vi "Demo for Ba RT.vi"(4 "Source:Advanced:Source Delay":dbl=4e-05 format="%#_6p", 5 "Source:Transient Response":i32(ring)=1039 items=["Slow"=1041, "Normal"=1038, "Fast"=1039, "Custom"=1042], 7 "Measurement:Sense":i32(ring)=1009 items=["Local"=1008, "Remote"=1009], 8 "channels":string="0", 9 "Current":dbl=0.4 format="%#_6p", 10 "Voltage":dbl=0.6 format="%#_6p", 11 "resource name":refnum<k15>="SMU") -> (2 "R":dbl=1.3110205691793813e-05 format="%#_8p")   [LabVIEW 2019]
uses:
  <instrlib>/niDCPower/nidcpower.llb/niDCPower Wait For Event - Event.ctl
  <vilib>/ptbypt/NI_PtbyPt.lvlib
panel:
  in  "Measurement:Aperture":dbl=0.0833333333333333 format="%#_6p"
  out "error out":errorcluster
  out "current measurements":dbl[](array[numeric])=[0.3999999270507816, -0.39999981518198563, -1.8644799301692494e-08]
  out "voltage measurements":dbl[](array[numeric])=[-3.375039148844662e-06, -1.386320032289827e-05, -8.551887933473147e-06]
  in  "Measurement:Advanced:DC Noise Rejection":i32(ring)=1044 items=["Normal"=1044, "Second-Order"=1043]
  in  "Source:Advanced:Sequence Loop Count":i32=100
  out "standard deviation":dbl=1.0179791126633813e-07 format="%.6p"
  out "Waveform Chart":dbl(graph)=1.3110205691793813e-05
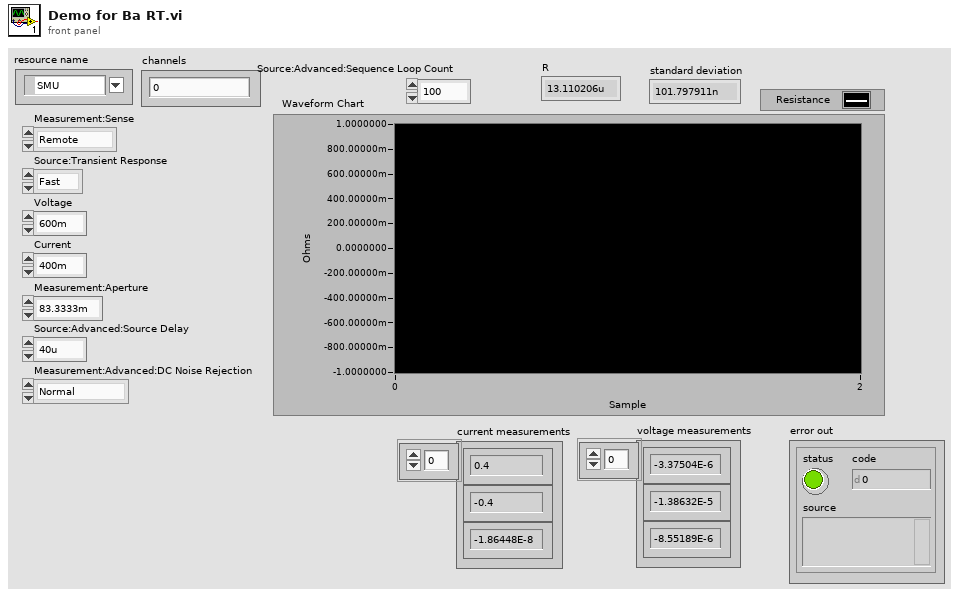
[diagram p1: front panel]
types:
  T1 = typedef "niDCPower Wait For Event - Event.ctl" = i32
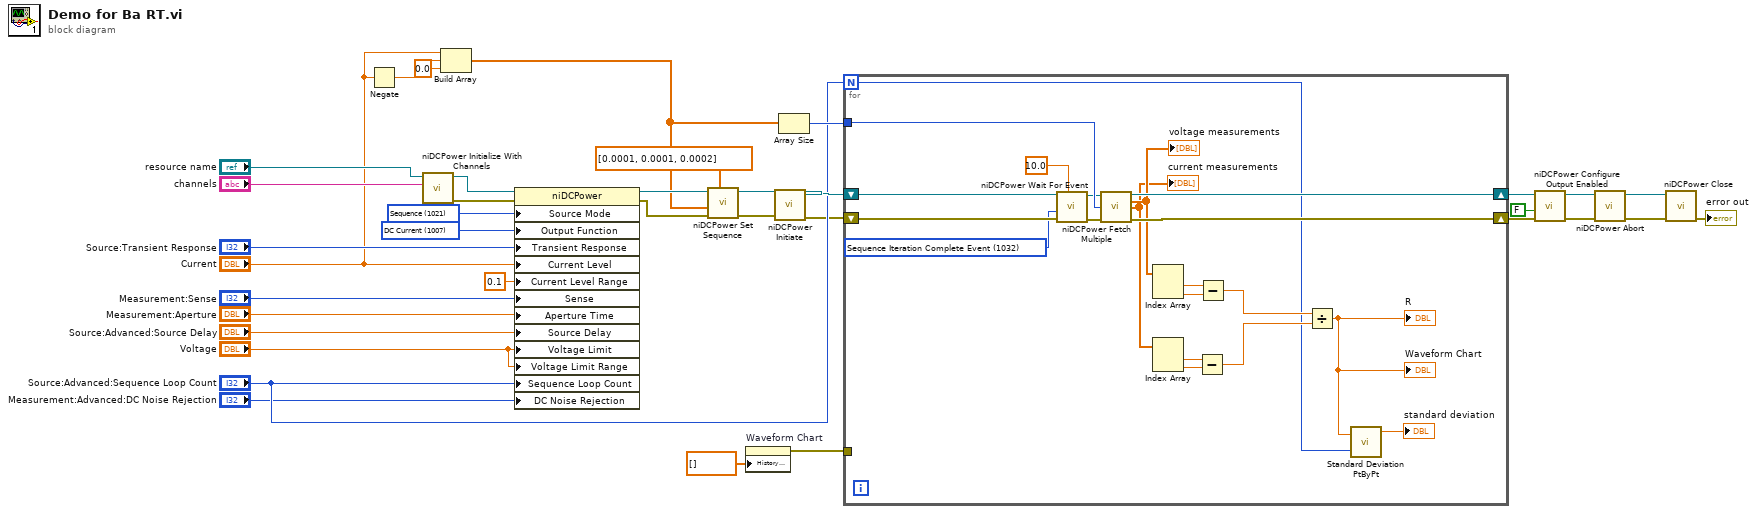
[diagram p0: block diagram]
diagram:
  w35 = 1007 items=["DC Voltage"=1006, "DC Current"=1007, "Pulse Voltage"=1049, "Pulse Current"=1050] ("Source:Output Function")
  w36 = 1021 items=["Single Point"=1020, "Sequence"=1021] ("Source:Source Mode")
  n1 = Negate(x="Current") -> (-x=w27:dbl)
  n2 = call <instrlib>:"niDCPower Initialize With Channels.vi"("channels"="channels", "resource name"="resource name") -> ("error out"=w22:errorcluster, "instrument handle out"=w23:refnum<k15>)  [unwired: 8 in]
  n3 = Build Array("Current", w27, 0.0 ("element")) -> (w26:dbl[])
  n4 = property class="niDCPower"(reference=w23, error in=w22, "Source Mode"=w36, "Output Function"=w35, "Transient Response"="Source:Transient Response", "Current Level"="Current", "Current Level Range"=0.1 ("Source:DC Current:Current Level Range"), "Sense"="Measurement:Sense", "Aperture Time"="Measurement:Aperture", "Source Delay"="Source:Advanced:Source Delay", "Voltage Limit"="Voltage", "Voltage Limit Range"="Voltage", "Sequence Loop Count"="Source:Advanced:Sequence Loop Count", "DC Noise Rejection"="Measurement:Advanced:DC Noise Rejection") -> (reference out=w31:refnum<k15>, error out=w32:errorcluster)
  n5 = call <instrlib>:"niDCPower Set Sequence.vi"("source delays"=dbl[] [0.0001, 0.0001, 0.0002], "error in (no error)"=w32, "values"=w26, "instrument handle"=w31) -> ("error out"=w4:errorcluster, "instrument handle out"=w29:refnum<k15>)  [unwired: 6 in]
  n6 = property on="Waveform Chart" class="WFChart (strict)"("History Data"=dbl[] []) -> (error out=w15:errorcluster)  [unwired: 2 in, 1 out]
  n7 = call <instrlib>:"niDCPower Initiate.vi"("error in (no error)"=w4, "instrument handle"=w29) -> ("error out"=w3:errorcluster, "instrument handle out"=w19:refnum<k15>)  [unwired: 8 in]
  n8 = Array Size(array=w26) -> (size(s)=w28:i32)
  n9 = for {
    N: "Source:Advanced:Sequence Loop Count" -> [w38]
    tunnel: w28 -> [w56]
    shift-right: [w48] -> w11
    shift-left: w3 -> [w55]
    shift-right: [w49] -> w12
    shift-left: w19 -> [w54]
    tunnel: w15 -> [_]
    w53 = T1 1032 items=["Source Complete Event"=1030, "Measure Complete Event"=1031, "Sequence Iteration Complete Event"=1032, "Sequence Engine Done Event"=1033, "Pulse Complete Event"=1051, "Ready For Pulse Trigger Event"=1052] ("event")
    n10 = call <instrlib>:"niDCPower Wait For Event.vi"("timeout (sec)"=10.0, "error in (no error)"=w55, "event"=w53, "instrument handle"=w54) -> ("error out"=w50:errorcluster, "instrument handle out"=w51:refnum<k15>)  [unwired: 6 in]
    n11 = call <instrlib>:"niDCPower Fetch Multiple.vi"("instrument handle"=w51, "count (1)"=w56, "error in (no error)"=w50) -> ("instrument handle out"=w49:refnum<k15>, "voltage measurements"=w47:dbl[], "current measurements"=w46:dbl[], "error out"=w48:errorcluster)  [unwired: 7 in, 2 out]
    "voltage measurements" <- w47
    "current measurements" <- w46
    n12 = Index Array(array=w47) -> (element #1=w45:dbl, element #2=w44:dbl)  [unwired: 2 in]
    n13 = Index Array(array=w46) -> (element #1=w42:dbl, element #2=w43:dbl)  [unwired: 2 in]
    n14 = Subtract(x=w42, y=w43) -> (x-y=w40:dbl)
    n15 = Subtract(x=w45, y=w44) -> (x-y=w41:dbl)
    n16 = Divide(x=w41, y=w40) -> (x/y=w39:dbl)
    "R" <- w39
    "Waveform Chart" <- w39
    n17 = call <vilib>:"Standard Deviation PtByPt.vi"("x"=w39, "sample length"=w38) -> ("standard deviation"=→"standard deviation":dbl)  [unwired: 1 in, 2 out]
  }
  n18 = call <instrlib>:"niDCPower Configure Output Enabled.vi"("error in (no error)"=w11, "output enabled"=FALSE, "instrument handle"=w12) -> ("error out"=w14:errorcluster, "instrument handle out"=w13:refnum<k15>)  [unwired: 7 in]
  n19 = call <instrlib>:"niDCPower Abort.vi"("error in (no error)"=w14, "instrument handle"=w13) -> ("error out"=w25:errorcluster, "instrument handle out"=w24:refnum<k15>)  [unwired: 8 in]
  n20 = call <instrlib>:"niDCPower Close.vi"("error in (no error)"=w25, "instrument handle"=w24) -> ("error out"=→"error out":errorcluster)  [unwired: 9 in]
